vi "DSF.Engine.Memory.Pointer.Channel Properties.New.vi"(8 "error in (no error)":errorcluster, 11 "count (1)":u64=1 format="%d elements") -> (0 "error out":errorcluster, 3 "Channel Properties pointer":refnum<class "DSF.Engine.Memory.Pointer.Channel Properties.lvclass">)   [LabVIEW 2016, in "DSF.Engine.lvlib" / "DSF.Engine.Memory.Pointer.Channel Properties.lvclass"]
uses:
  DSF.Engine.Memory.Pointer.Channel Properties.lvclass
  C:/Git/SourceTree/DSF/Source/Classes/Memory.Pointer.Array/DSF.Engine.Memory.Pointer.Array.lvclass
  Typedefs/DSF.Shared.Channel Configuration.ctl
  Typedefs/DSF.Shared.Data Type.ctl
  DSF.Shared.lvlib
  Memory.Pointer.Array/DSF.Engine.Memory.Pointer.Array.lvclass
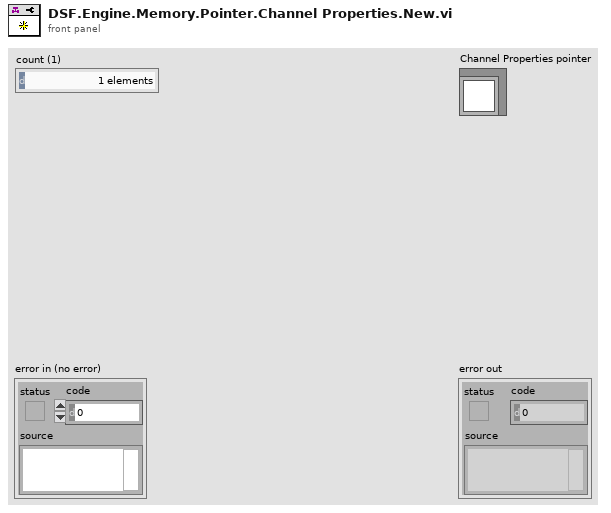
[diagram p1: front panel]
types:
  T1 = typedef "DSF.Shared.lvlib/DSF.Shared.Channel Configuration.ctl" = cluster{"data type":T2, "offset":u64, "size":u64, "count":u64}
  T2 = typedef "DSF.Shared.lvlib/DSF.Shared.Data Type.ctl" = enum8{"Bool", "SGL", "DBL", "I8", "I16", "I32", "I64", "U8", "U16", "U32", "U64"}
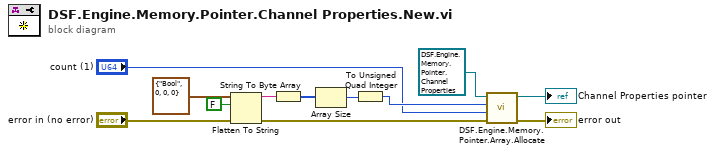
[diagram p0: block diagram]
diagram:
  n1 = Flatten To String(anything=T1 {"data type"=enum."Bool", "offset"=0, "size"=0, "count"=0} ("Channel properties"), prepend array or string size? (T)=FALSE, error in (no error)="error in (no error)") -> (data string=w9:string, error out=w6:errorcluster)  [unwired: 1 in, 1 out]
  n2 = String To Byte Array(string=w9) -> (unsigned byte array=w8:u8[])
  n3 = Array Size(array=w8) -> (size(s)=w7:i32)
  n4 = To Unsigned Quad Integer(1:w7) -> (0:w5:u64)
  n5 = call "DSF.Engine.Memory.Pointer.Array.Allocate.vi"("error in (no error)"=w6, "count (1)"="count (1)", "element size"=w5, "Array Pointer in"=refnum<class "DSF.Engine.Memory.Pointer.Channel Properties.lvclass"> refnum ("Channel Properties pointer")) -> ("error out"=→"error out":errorcluster, "Array Pointer out"=→"Channel Properties pointer":refnum<class "DSF.Engine.Memory.Pointer.Channel Properties.lvclass">)  [unwired: 6 in]
